vi "Histogram_Main Function.vi"(6 "ROI Descriptor":T1 {"Contours"."Type" items=["No Selection", "Point", "Line", "Rectangle", "Oval", "Polygon", "Free", "Annulus", "Unused2", "Unused3", "Broken Line", "Free Hand Line", "Rotated Rectangle"]}, 7 "Number of Classes":i32=256, 8 "error in (no error)":errorcluster, 9 "Image Mask":T2, 10 "Interval Range":cluster{"Minimum":sgl, "Maximum":sgl} {"Maximum" format="%.2f"; "Minimum" format="%.2f"}, 11 "Refnum in":T2) -> (0 "error out":errorcluster, 2 "Histogram Report":T3 {"Standard  Variation" format="%.2f"; "Mean Value" format="%.2f"; "Interval Width" format="%.2f"; "Starting Value" format="%.2f"; "Maximal Value" format="%.2f"; "Minimal Value" format="%.2f"}, 3 "Refnum out":T2)   [LabVIEW 2019]
uses:
  <vilib>/vision/Image Controls.llb/IMAQ Image.ctl
  <vilib>/vision/NI_Vision_Development_Module.lvlib
panel:
  out "Image":T2(plugin-control)
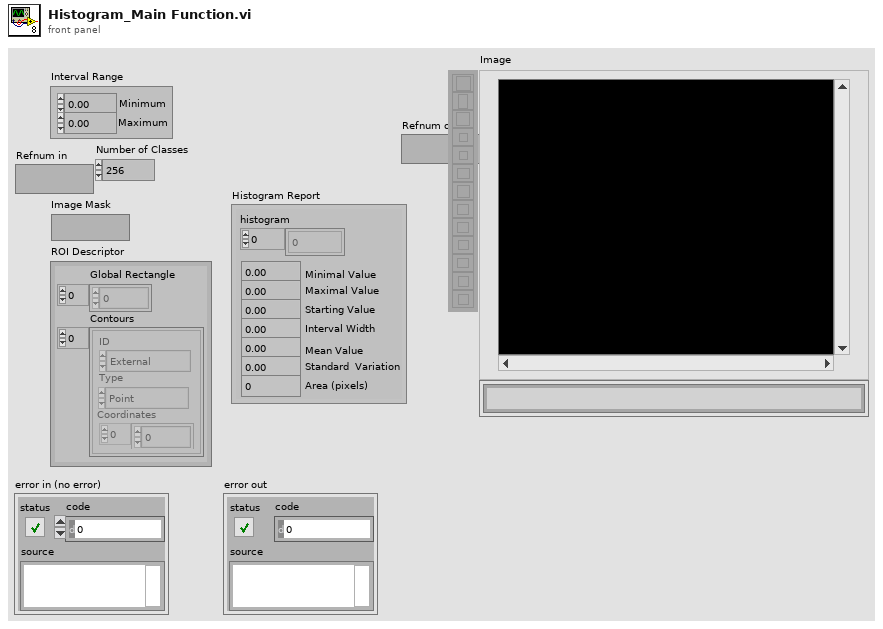
[diagram p1: front panel]
types:
  T1 = cluster{"Global Rectangle":i32[], "Contours":cluster{"ID":enum32{"External", "Internal"}, "Type":u32, "Coordinates":i32[]}[]}
  T2 = typedef "IMAQ Image.ctl" = refnum<image>
  T3 = cluster{"histogram":u32[], "Minimal Value":sgl, "Maximal Value":sgl, "Starting Value":sgl, "Interval Width":sgl, "Mean Value":sgl, "Standard  Variation":sgl, "Area (pixels)":i32}
  T4 = cluster{"Minimal Value":sgl, "Maximal Value":sgl, "Mean Value":sgl, "Standard  Variation":sgl, "Area (pixels)":i32}
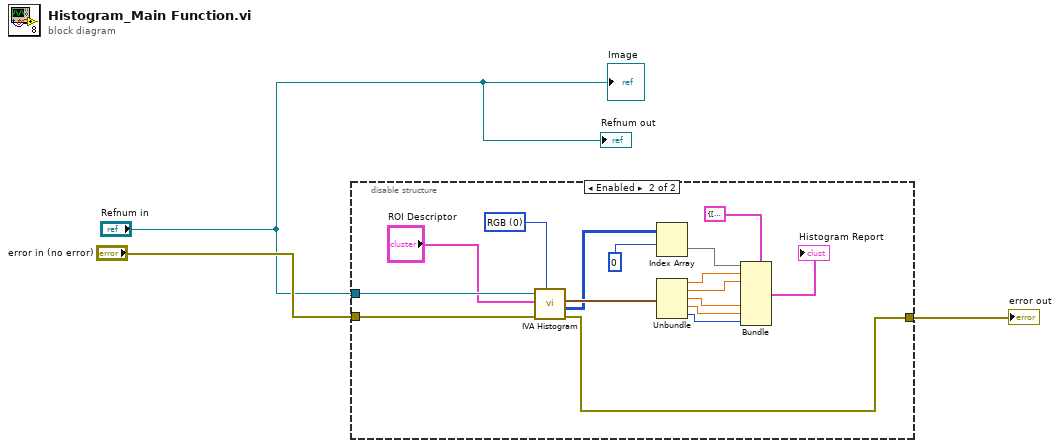
[diagram p0: block diagram]
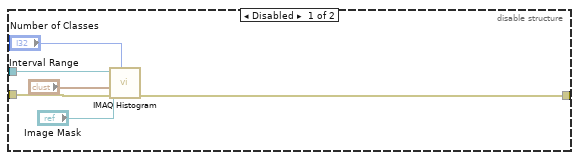
[diagram p2: hidden frame]
diagram:
  n1 = disable-structure shown="Enabled" {
    disable-tunnel: [w9 w22] -> w3
    disable-tunnel: "error in (no error)" -> [w8 w23]
    disable-tunnel: "Refnum in" -> [w4 w24]
    frame Disabled {
      n2 = call "IMAQ Histogram"("Number of Classes"="Number of Classes", "error in (no error)"=w8, "Interval Range"="Interval Range", "Image Mask"="Image Mask", "Image"=w4) -> ("error out"=w9:errorcluster)  [unwired: 5 in, 1 out]
    }
    frame Enabled {
      w25 = u16 0 items=["RGB", "HSL", "HSV", "HSI"] ("Color Mode")
      n3 = call <vilib>:"IVA Histogram.vi"("Color Mode"=w25, "error in (no error)"=w23, "ROI Descriptor"="ROI Descriptor", "Image In"=w24) -> ("error out"=w22:errorcluster, "Histograms"=w19:u32[][], "Statistics"=w21:T4)  [unwired: 5 out]
      n4 = Index Array(array=w19, index (row)=0) -> (element=w17:u32[])  [unwired: 1 in]
      n5 = Unbundle(w21) -> ("Minimal Value"=w16:sgl, "Maximal Value"=w15:sgl, "Mean Value"=w14:sgl, "Standard  Variation"=w13:sgl, "Area (pixels)"=w12:i32)
      n6 = Bundle(cluster=T3 {"histogram"=[782, 0, 0, 0, 0, 0, 0, 0, 0, 0, 0, 0, 0, 0, 0, 0, 0, 0, 0, 0, 0, 0, 0, 0, 0, 0, 0, 0, 0, 0, 0, 0, 0, 0, 0, 0, 0, 0, 0, 0, 0, 0, 0, 0, 0, 0, 0, 0, 0, 0, 0, 0, 0, 0, 0, 0, 0, 0, 0, 0, 0, 0, 0, 0, 0, 0, 0, 0, 0, 0, 0, 0, 0, 0, 0, 0, 0, 0, 0, 0, 0, 0, 0, 0, 0, 0, 0, 0, 0, 0, 0, 0, 0, 0, 0, 0, 0, 0, 0, 0, 0, 0, 0, 0, 0, 0, 0, 0, 0, 0, 0, 0, 0, 0, 0, 0, 0, 0, 0, 0, 0, 0, 0, 0, 0, 0, 0, 0, 0, 0, 0, 0, 0, 0, 0, 0, 0, 0, 0, 0, 0, 0, 0, 0, 0, 0, 0, 0, 0, 0, 0, 0, 0, 0, 0, 0, 0, 0, 0, 0, 0, 0, 0, 0, 0, 0, 0, 0, 0, 0, 0, 0, 0, 0, 0, 0, 0, 0, 0, 0, 0, 0, 0, 0, 0, 0, 0, 0, 0, 0, 0, 0, 0, 0, 0, 0, 0, 0, 0, 0, 0, 0, 0, 0, 0, 0, 0, 0, 0, 0, 0, 0, 0, 0, 0, 0, 0, 0, 0, 0, 0, 0, 0, 0, 0, 0, 0, 0, 0, 0, 0, 0, 0, 0, 0, 0, 0, 0, 0, 0, 0, 0, 0, 0, 0, 0, 0, 0, 0, 0, 0, 0, 0, 0, 0, 0], "Minimal Value"=0.0, "Maximal Value"=0.0, "Starting Value"=0.0, "Interval Width"=1.0, "Mean Value"=0.0, "Standard  Variation"=0.0, "Area (pixels)"=782} ("Histogram Report"), "histogram"=w17, "Minimal Value"=w16, "Maximal Value"=w15, "Mean Value"=w14, "Standard  Variation"=w13, "Area (pixels)"=w12) -> (→"Histogram Report":T3)  [unwired: 2 in]
    }
  }
  "error out" <- w3
  "Refnum out" <- "Refnum in"
  "Image" <- "Refnum in"
